vi "time_display.vi"(9 "scan map in":T1, 10 "test start time":u32, 11 "millisecond timer value":u32) -> (2 "estimated time remaining":string, 3 "elapsed time":string)   [LabVIEW 2011]
uses:
  <vilib>/vision/Image Controls.llb/IMAQ Image.ctl
  <vilib>/Utility/error.llb/DialogType.ctl
  <vilib>/vision/NI_Vision_Development_Module.lvlib
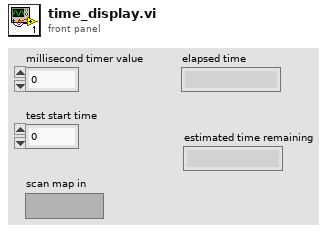
[diagram p1: front panel]
types:
  T1 = typedef "IMAQ Image.ctl" = refnum<image>
  T2 = typedef "DialogType.ctl" = u16
  T3 = cluster{"Mean Value":sgl, "Standard Variation":sgl, "Minimal Value":sgl, "Maximal Value":sgl, "Area (calibrated)":sgl, "Area (pixels)":u32, "%":sgl, "Calibration Valid":bool}
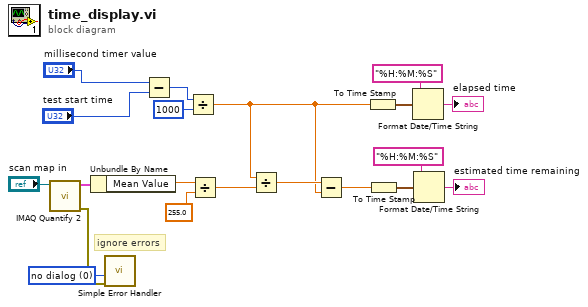
[diagram p0: block diagram]
diagram:
  w5 = T2 0 items=["no dialog", "OK message", "continue or stop message", "OK message + warnings", "continue/stop + warnings"] ("type of dialog (OK msg:1)")
  # "ignore errors"
  n1 = call "IMAQ Quantify 2"("Image"="scan map in") -> ("error out"=w6:errorcluster, "Global Report"=w12:T3)  [unwired: 8 in, 1 out]
  n2 = Unbundle By Name(w12) -> ("Mean Value"=w8:sgl)
  n3 = call <vilib>:"Simple Error Handler.vi"("type of dialog (OK msg:1)"=w5, "error in (no error)"=w6) -> ()  [unwired: 3 in, 5 out]
  n4 = Subtract(x="millisecond timer value", y="test start time") -> (x-y=w15:u32)
  n5 = Divide(x=w15, y=u32 1000) -> (x/y=w2:dbl)
  n6 = Divide(x=w8, y=sgl 255.0) -> (x/y=w4:sgl)
  n7 = Divide(x=w2, y=w4) -> (x/y=w3:dbl)
  n8 = Subtract(x=w3, y=w2) -> (x-y=w1:dbl)
  n9 = To Time Stamp(1:w2) -> (0:w17:timestamp)
  n10 = To Time Stamp(1:w1) -> (0:w11:timestamp)
  n11 = Format Date/Time String(time format string (%c)="%H:%M:%S", seconds (now)=w17) -> (date/time string=→"elapsed time":string)  [unwired: 1 in]
  n12 = Format Date/Time String(time format string (%c)="%H:%M:%S", seconds (now)=w11) -> (date/time string=→"estimated time remaining":string)  [unwired: 1 in]
